vi "FTW-Actor-Subscription-Add.vi"(0 "FTW-ActorInstance In":refnum<class "FTW-ActorInstance.lvclass">, 5 "Subscriber Name":string, 7 "Subscriber URI":string, 9 "Connection Timeout":i32=100 caption="Connection Timeout (100 ms)" format="%d ms", 11 "error in":errorcluster) -> (4 "FTW-ActorInstance Out":refnum<class "FTW-ActorInstance.lvclass">, 15 "error out":errorcluster)   [LabVIEW 2015, in "FTW-ActorInstance.lvclass"]
uses:
  FTW-ActorInstance.lvclass
  FTW-ActorInstance.lvclass/FTW-ActorInstance.ctl
  Subscriber/FTW-Subscriber.lvclass
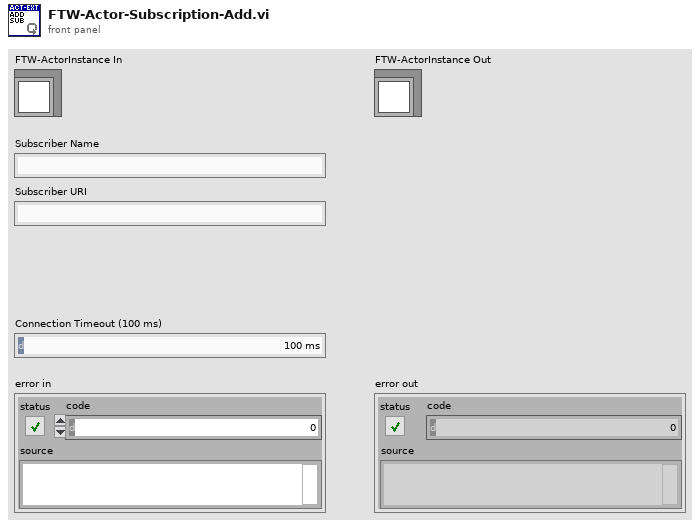
[diagram p1: front panel]
types:
  T1 = cluster{"Subscriber Name":string, "Subscriber URI":string}
  T2 = cluster{"Subscriber Name":string, "Subscriber URI":string}[]
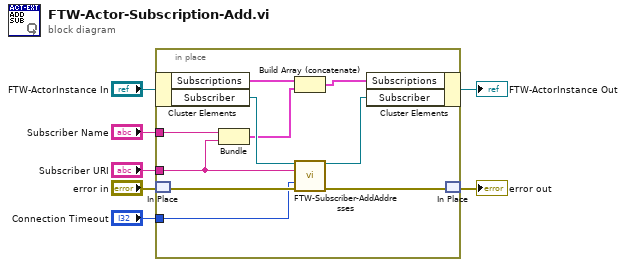
[diagram p0: block diagram]
diagram:
  n1 = in-place {
    in-place-border: "Subscriber URI" -> [w12]
    in-place-border: "Subscriber Name" -> [w13]
    in-place-border: "Connection Timeout" -> [w8]
    n2 = in-place-cluster #1("FTW-ActorInstance In") -> ("Subscriptions"=w9:cluster{"Name":string, "URI":string}[], "Subscriber"=w17:refnum<class "FTW-Subscriber.lvclass">)
    n3 = in-place-match #2("error in") -> (w15:errorcluster)
    n4 = Bundle("Subscriber Name"=w13, "Subscriber URI"=w12) -> (w11:T1)  [unwired: 1 in]
    n5 = Build Array (concatenate)(w9, w11) -> (w10:T2)
    n6 = call "FTW-Subscriber-AddAddresses.vi"("FTW-Subscription In"=w17, "Addresses"=w12, "Connection Timeout"=w8, "error in"=w15) -> ("FTW-Subscription Out"=w16:refnum<class "FTW-Subscriber.lvclass">, "error out"=w14:errorcluster)  [unwired: 10 in]
    n7 = in-place-cluster #1("Subscriptions"=w10, "Subscriber"=w16) -> (→"FTW-ActorInstance Out":refnum<class "FTW-ActorInstance.lvclass">)
    n8 = in-place-match #2(w14) -> (→"error out":errorcluster)
  }
